vi "Cooler OFF.vi"(8 "error in (no error)":errorcluster, 11 "Cooler.lvclass":refnum<class "Cooler.lvclass">) -> (0 "error out":errorcluster, 3 "Cooler.lvclass":refnum<class "Cooler.lvclass">)   [LabVIEW 2018, in "Cooler.lvclass"]
uses:
  Cooler/Cooler.lvclass
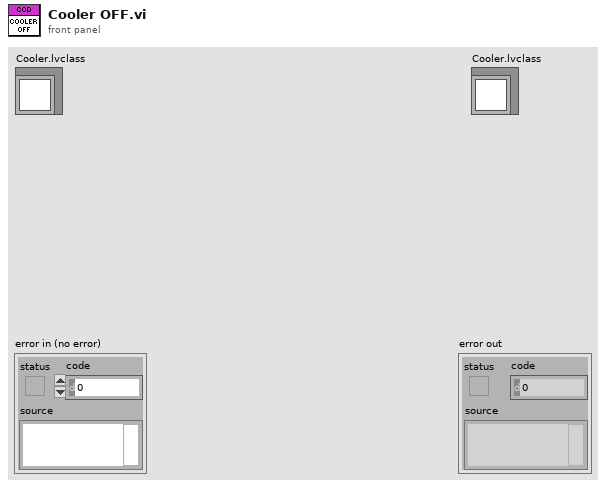
[diagram p1: front panel]
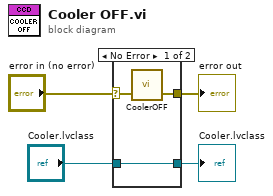
[diagram p0: block diagram]
diagram:
  n1 = case shown="No Error" "error in (no error)" {
    selector: "error in (no error)" -> [w6 w9]
    tunnel: [w5 w9] -> w3
    tunnel: [w7 w8] -> w1
    tunnel: "Cooler.lvclass" -> [w7 w8]
    frame No Error {
      n2 = call <userlib>:"CoolerOFF.vi"("error in (no error)"=w6) -> ("error out"=w5:errorcluster)  [unwired: 1 in, 1 out]
    }
    frame Error {
    }
  }
  "error out" <- w3
  "Cooler.lvclass" <- w1
